vi "ReadFIFOs.vi"(0 "FPGA In":T1, 2 "Error In":errorcluster, 3 "Trap N Read":u32, 4 "APD N Read":u32, 5 "TPos N Read":u32) -> (10 "FPGA Out":T1, 12 "Error Out":errorcluster, 14 "Trap Data":i16[](array[numeric]), 15 "APD Data":u32[](array[numeric]), 16 "TPos Data":u64[](array[numeric]), 17 "Trap N Left":u32, 18 "APD N Left":u32, 19 "TPos N Left":u32)   [LabVIEW 2013]
uses:
  openfpgaref.8.6.ctl
  <vilib>/rvi/interface/common/niFpgaWaitOnOcc.vi
  <vilib>/Utility/error.llb/Error Cluster From Error Code.vi
  <vilib>/rvi/errors/niLvFpgaAdjustHostInterfaceError.vi
  <vilib>/rvi/interface/nirviMethod/nirviMethod.xnode
  FPGA Bitfiles/UHR-FleezersInst_FPGATarget_UHR-FleezersCont_IqK95Pvv9lYv5.3.lvbitx
  <vilib>/FPGAPlugInAG/PCIe-7852R/niLvFpga_ReadFifo_PCIe-7852R.vi
  <vilib>/rvi/errors/niLvFpgaMergeErrorWithErrorCode.vi
panel:
  # "DONT USE - FIFO Read cannot be inlined"
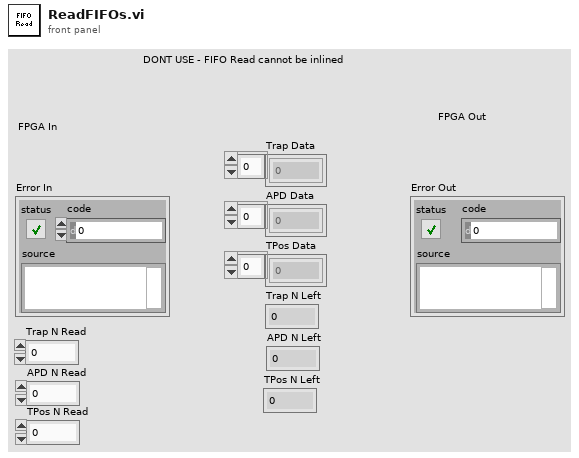
[diagram p1: front panel]
types:
  T1 = typedef "openfpgaref.8.6.ctl" = refnum<k20>
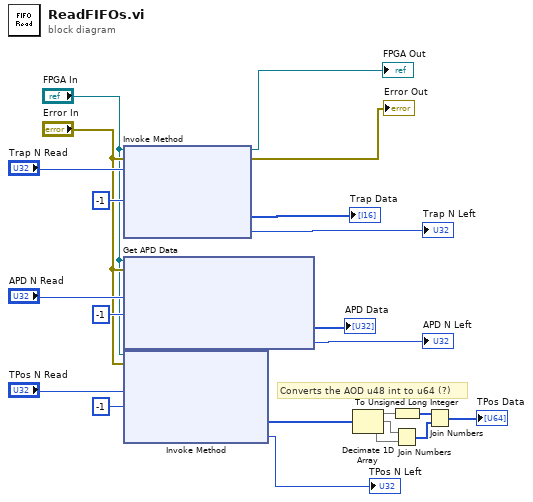
[diagram p0: block diagram]
diagram:
  # "Converts the AOD u48 int to u64 (?)"
  n1 = xnode "Invoke Method"("FPGA VI Reference In"="FPGA In", "error in"="Error In", "Number of Elements"="Trap N Read", "Timeout (ms)"=-1 ("Timeout")) -> ("FPGA VI Reference Out"=→"FPGA Out":T1, "error out"=→"Error Out":errorcluster, "Data"=→"Trap Data":i16[], "Elements Remaining"=→"Trap N Left":u32)
  n2 = xnode "Get APD Data"("FPGA VI Reference In"="FPGA In", "error in"="Error In", "Number of Elements"="APD N Read", "Timeout (ms)"=-1) -> ("Data"=→"APD Data":u32[], "Elements Remaining"=→"APD N Left":u32)  [unwired: 2 out]
  n3 = xnode "Invoke Method"("FPGA VI Reference In"="FPGA In", "error in"="Error In", "Number of Elements"="TPos N Read", "Timeout (ms)"=-1) -> ("Data"=w10:u16[], "Elements Remaining"=→"TPos N Left":u32)  [unwired: 2 out]
  n4 = Decimate 1D Array(w10) -> (w12:u16[], w11:u16[], w3:u16[])
  n5 = To Unsigned Long Integer(number=w12) -> (unsigned 32bit integer=w13:u32[])
  n6 = Join Numbers(hi=w11, lo=w3) -> ((hi.lo)=w14:u32[])
  n7 = Join Numbers(hi=w13, lo=w14) -> ((hi.lo)=→"TPos Data":u64[])
